vi "Generate PWM.vi"(9 "Connector m Bank n PWM Generation Settings":T1={"PWM 0 Settings"={"ACTIVE EDGE"=TRUE, "ACTIVE TICKS"=0, "INACTIVE TICKS"=0}, "PWM 1 Settings"={"ACTIVE EDGE"=TRUE, "ACTIVE TICKS"=0, "INACTIVE TICKS"=0}, "PWM 2 Settings"={"ACTIVE EDGE"=TRUE, "ACTIVE TICKS"=0, "INACTIVE TICKS"=0}, "PWM 3 Settings"={"ACTIVE EDGE"=TRUE, "ACTIVE TICKS"=0, "INACTIVE TICKS"=0}, "PWM 4 Settings"={"ACTIVE EDGE"=TRUE, "ACTIVE TICKS"=0, "INACTIVE TICKS"=0}, "PWM 5 Settings"={"ACTIVE EDGE"=TRUE, "ACTIVE TICKS"=0, "INACTIVE TICKS"=0}, "PWM 6 Settings"={"ACTIVE EDGE"=TRUE, "ACTIVE TICKS"=0, "INACTIVE TICKS"=0}, "PWM 7 Settings"={"ACTIVE EDGE"=TRUE, "ACTIVE TICKS"=0, "INACTIVE TICKS"=0}}, 11 "Bank in":refnum<class "Bank.lvclass">) -> (3 "Bank out":refnum<class "Bank.lvclass">)   [LabVIEW 2019, in "LRUTS FPGA IP.lvlib" / "Bank.lvclass"]
uses:
  Bank.lvclass
  PWM Generation Bank Settings.ctl
  PWM Generation Channel Settings.ctl
  Bank Type.ctl
  Bank.lvclass/Bank.ctl
  <vilib>/rvi/eio/common/nirviEmuTemplateMethod_errors.vi
  <vilib>/eio/EIONode/EIONode.xnode
  <instrlib>/_niInstr/Basic Elements/v1/FPGA/niInstr Basic Elements v1 FPGA.lvlib
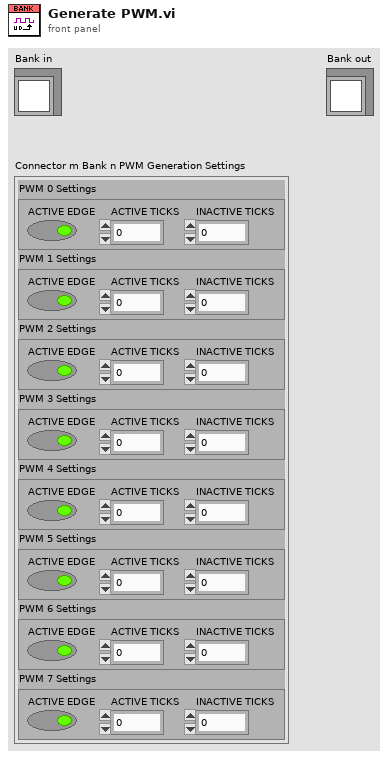
[diagram p1: front panel]
types:
  T1 = typedef "LRUTS FPGA IP.lvlib/Bank.lvclass/PWM Generation Bank Settings.ctl" = cluster{"PWM 0 Settings":T2, "PWM 1 Settings":T2, "PWM 2 Settings":T2, "PWM 3 Settings":T2, "PWM 4 Settings":T2, "PWM 5 Settings":T2, "PWM 6 Settings":T2, "PWM 7 Settings":T2}
  T2 = typedef "LRUTS FPGA IP.lvlib/Bank.lvclass/PWM Generation Channel Settings.ctl" = cluster{"ACTIVE EDGE":bool, "ACTIVE TICKS":u32, "INACTIVE TICKS":u32}
  T3 = typedef "LRUTS FPGA IP.lvlib/Bank.lvclass/Bank Type.ctl" = enum16{"None", "Discrete Acquisition", "Discrete Generation", "PWM Acquisition", "PWM Generation"}
  T4 = typedef "LRUTS FPGA IP.lvlib/Bank.lvclass/FPGA IO Resources.ctl" = cluster{"DIO 0":refnum<k21>, "DIO 1":refnum<k21>, "DIO 2":refnum<k21>, "DIO 3":refnum<k21>, "DIO 4":refnum<k21>, "DIO 5":refnum<k21>, "DIO 6":refnum<k21>, "DIO 7":refnum<k21>}
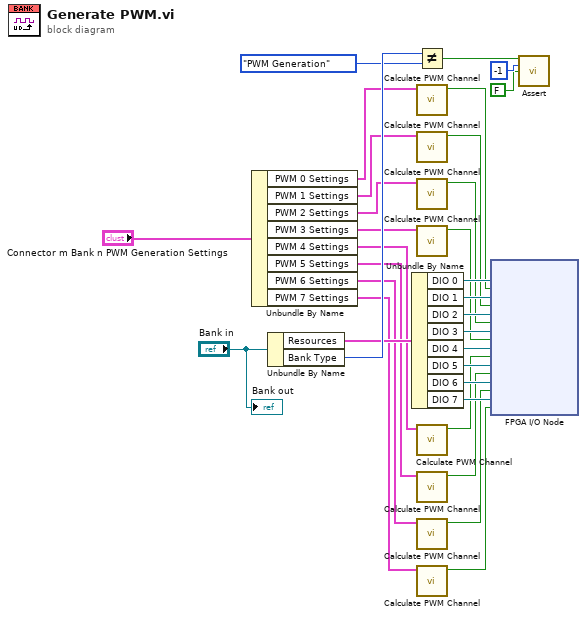
[diagram p0: block diagram]
diagram:
  n1 = Unbundle By Name("Connector m Bank n PWM Generation Settings") -> ("PWM 0 Settings"=w16:T2, "PWM 1 Settings"=w15:T2, "PWM 2 Settings"=w14:T2, "PWM 3 Settings"=w13:T2, "PWM 4 Settings"=w12:T2, "PWM 5 Settings"=w11:T2, "PWM 6 Settings"=w10:T2, "PWM 7 Settings"=w9:T2)
  n2 = Unbundle By Name("Bank in") -> ("Resources"=w26:T4, "Bank Type"=w31:T3)
  n3 = Unbundle By Name(w26) -> ("DIO 0"=w25:refnum<k21>, "DIO 1"=w24:refnum<k21>, "DIO 2"=w23:refnum<k21>, "DIO 3"=w22:refnum<k21>, "DIO 4"=w21:refnum<k21>, "DIO 5"=w20:refnum<k21>, "DIO 6"=w19:refnum<k21>, "DIO 7"=w18:refnum<k21>)
  n4 = Not Equal?(x=w31, y=Bank_Type."PWM Generation") -> (x != y?=w29:bool)
  n5 = call "Calculate PWM Channel.vi"("Settings"=w16) -> ("Output"=w8:bool)  [unwired: 10 in]
  n6 = call "Calculate PWM Channel.vi"("Settings"=w15) -> ("Output"=w7:bool)  [unwired: 10 in]
  n7 = call "Calculate PWM Channel.vi"("Settings"=w14) -> ("Output"=w6:bool)  [unwired: 10 in]
  n8 = call "Calculate PWM Channel.vi"("Settings"=w13) -> ("Output"=w5:bool)  [unwired: 10 in]
  n9 = call "Calculate PWM Channel.vi"("Settings"=w12) -> ("Output"=w4:bool)  [unwired: 10 in]
  n10 = call "Calculate PWM Channel.vi"("Settings"=w11) -> ("Output"=w3:bool)  [unwired: 10 in]
  n11 = call "Calculate PWM Channel.vi"("Settings"=w10) -> ("Output"=w2:bool)  [unwired: 10 in]
  n12 = call "Calculate PWM Channel.vi"("Settings"=w9) -> ("Output"=w1:bool)  [unwired: 10 in]
  n13 = xnode "FPGA I/O Node"("I/O Item"=w8, "FPGA I/O In"=w25, "I/O Item"=w7, "FPGA I/O In"=w24, "I/O Item"=w6, "FPGA I/O In"=w23, "I/O Item"=w5, "FPGA I/O In"=w22, "I/O Item"=w4, "FPGA I/O In"=w21, "I/O Item"=w3, "FPGA I/O In"=w20, "I/O Item"=w2, "FPGA I/O In"=w19, "I/O Item"=w1, "FPGA I/O In"=w18) -> ()  [unwired: 8 out]
  n14 = call <instrlib>:"Assert.vi"("assert"=w29, "error code"=-1, "enable show error"=FALSE) -> ()  [unwired: 13 in]
  "Bank out" <- "Bank in"
